vi "Notify.vi"(8 "error in (no error)":errorcluster, 9 "Kill notifier":bool, 10 "Message":string, 11 "Mag Lab Root in":refnum<class "Mag Lab Root.lvclass">) -> (0 "error out":errorcluster, 3 "Mag Lab Root out":refnum<class "Mag Lab Root.lvclass">)   [LabVIEW 2015, in "Mag Lab Root.lvclass"]
uses:
  Mag Lab Root.lvclass
  Mag Lab Root.lvclass/Mag Lab Root.ctl
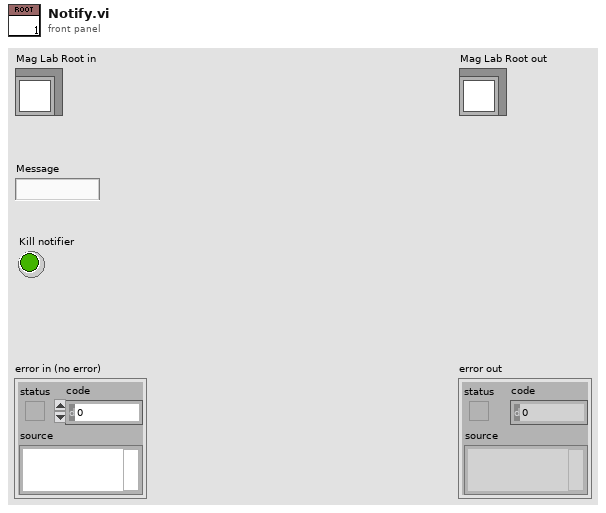
[diagram p1: front panel]
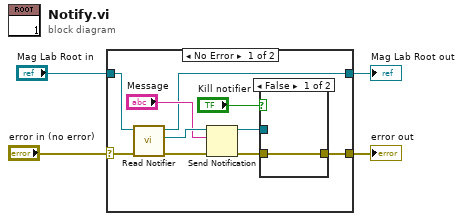
[diagram p0: block diagram]
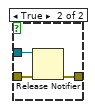
[diagram p2: hidden frame]
diagram:
  n1 = case shown="No Error" "error in (no error)" {
    selector: "error in (no error)" -> [w11 w20]
    tunnel: [w6 w20] -> w3
    tunnel: [w5 w19] -> w1
    tunnel: "Mag Lab Root in" -> [w14 w19]
    frame No Error {
      n2 = call "Read Notifier.vi"("error in (no error)"=w11, "Mag Lab Root in"=w14) -> ("error out"=w10:errorcluster, "Notifier"=w13:refnum<notifier>, "Mag Lab Root out"=w5:refnum<class "Mag Lab Root.lvclass">)  [unwired: 7 in]
      n3 = Send Notification(notification="Message", notifier=w13, error in (no error)=w10) -> (notifier out=w7:refnum<notifier>, error out=w8:errorcluster)
      n4 = case shown="False" "Kill notifier" {
        tunnel: w8 -> [w15 w18]
        tunnel: w7 -> [_ w17]
        tunnel: [w15 w16] -> w6
        frame False {
        }
        frame True {
          n5 = Release Notifier(notifier=w17, error in (no error)=w18) -> (error out=w16:errorcluster)  [unwired: 1 in, 2 out]
        }
      }
    }
    frame Error {
    }
  }
  "error out" <- w3
  "Mag Lab Root out" <- w1
